vi "Image Averaging Grab (SubVI).vi"(8 "error in":errorcluster, 10 "Number of Samples":i32, 11 "Camera Session In":T1) -> (0 "error out":errorcluster, 3 "Avg Image":T2(plugin-control))   [LabVIEW 2016]
doc: "The Snap VI acquires an image and displays the image in an image control using low-level acquisition VIs. A snap is appropriate for low-speed or single-capture applications in which ease of programming is essential."
uses:
  <vilib>/userdefined/High Color/IMAQdx.ctl
  <vilib>/vision/driver/NI_Vision_Acquisition_Software.lvlib
  <resource>/objmgr/IMAQImage.rc
panel:
  in  "Standalone Mode":bool
  out "Sample #":i32
  in  "Camera Name":refnum<k21> caption="IMAQdx Session"
  out "Image":T2(plugin-control)
  # "Overview: Creates an average image from a set of collected images.\nRequirements: Vision Acquisition Software\nInstructions: \n1. Select the Camera Name.\n2. Run the VI"
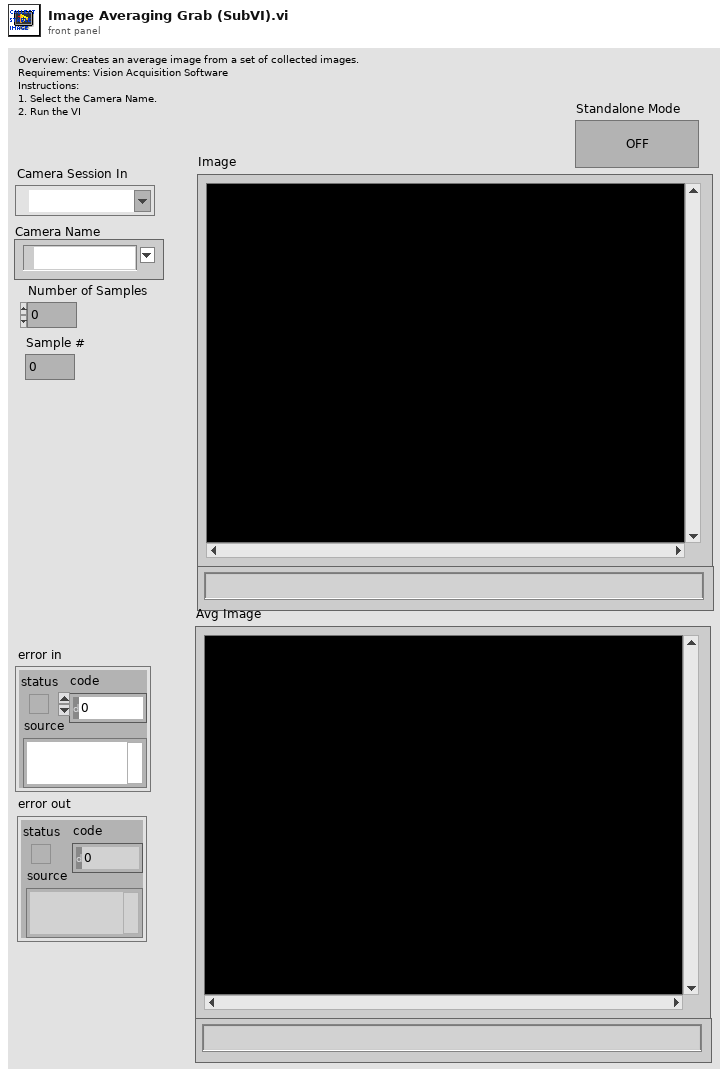
[diagram p1: front panel]
types:
  T1 = typedef "IMAQdx.ctl" = refnum<k21>
  T2 = typedef "IMAQ Image.ctl" = refnum<image>
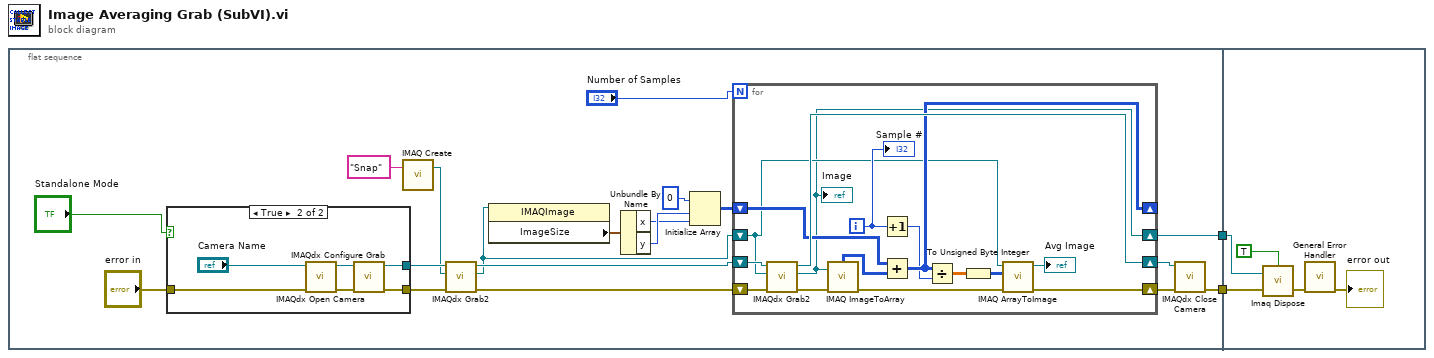
[diagram p0: block diagram]
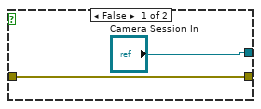
[diagram p2: hidden frame]
diagram:
  n1 = flat-sequence {
    tunnel: [w20] -> w2
    tunnel: [w9] -> w1
    tunnel: w2 -> [w50]
    tunnel: w1 -> [w48]
    frame #0 {
      n2 = case shown="True" "Standalone Mode" {
        tunnel: ["Camera Session In" w27] -> w13
        tunnel: [w22 w26] -> w11
        tunnel: "error in" -> [w22 w25]
        frame False {
        }
        frame True {
          n3 = call <vilib>:"IMAQdx Open Camera.vi"("error in"=w25, "Session In"="Camera Name") -> ("error out"=w28:errorcluster, "Session Out"=w29:T1)  [unwired: 1 in, 7 out]
          n4 = call <vilib>:"IMAQdx Configure Grab.vi"("error in"=w28, "Session In"=w29) -> ("error out"=w26:errorcluster, "Session Out"=w27:T1)  [unwired: 8 out]
        }
      }
      n5 = call "IMAQ Create"("Image Name"="Snap") -> ("New Image"=w12:T2)  [unwired: 3 in, 2 out]
      n6 = call <vilib>:"IMAQdx Grab2.vi"("error in"=w11, "Image In"=w12, "Session In"=w13) -> ("error out"=w8:errorcluster, "Image Out"=w7:T2, "Session Out"=w10:T1)  [unwired: 5 in, 1 out]
      n7 = property class="IMAQImage"(reference=w7) -> ("ImageSize"=w16:cluster{"x":i32, "y":i32})  [unwired: 1 in, 2 out]
      n8 = Unbundle By Name(w16) -> ("x"=w5:i32, "y"=w6:i32)
      n9 = Initialize Array(0 ("element"), w6, w5) -> (w15:i32[][])
      n10 = for {
        N: "Number of Samples" -> [_]
        shift-right: [w45] -> w21
        shift-left: w10 -> [w44]
        shift-right: [w33] -> w18
        shift-left: w8 -> [w43]
        shift-right: [w39] -> _
        shift-left: w15 -> [w40]
        shift-right: [w30] -> w9
        shift-left: w7 -> [w31]
        i -> [w38]
        n11 = call <vilib>:"IMAQdx Grab2.vi"("error in"=w43, "Image In"=w31, "Session In"=w44) -> ("error out"=w42:errorcluster, "Image Out"=w30:T2, "Session Out"=w45:T1)  [unwired: 5 in, 1 out]
        "Image" <- w30
        n12 = call "IMAQ ImageToArray"("error in (no error)"=w42, "Image"=w30) -> ("error out"=w34:errorcluster, "Image Pixels (U8)"=w41:u8[][])  [unwired: 2 in, 3 out]
        n13 = Increment(x=w38) -> (x+1=w37:i32)
        n14 = Add(x=w40, y=w41) -> (x+y=w39:i32[][])
        n15 = Divide(x=w39, y=w37) -> (x/y=w36:dbl[][])
        n16 = To Unsigned Byte Integer(number=w36) -> (unsigned 8bit integer=w35:u8[][])
        n17 = call "IMAQ ArrayToImage"("error in (no error)"=w34, "Image Pixels (U8)"=w35, "Image"=w31) -> ("error out"=w33:errorcluster, "Image Out"=→"Avg Image":T2)  [unwired: 7 in]
        "Sample #" <- w38
      }
      n18 = call <vilib>:"IMAQdx Close Camera.vi"("error in"=w18, "Session In"=w21) -> ("error out"=w20:errorcluster)  [unwired: 9 out]
    }
    frame #1 {
      n19 = call "Imaq Dispose"("All Images? (No)"=TRUE, "Image"=w48, "error in (no error)"=w50) -> ("error out"=w49:errorcluster)  [unwired: 3 in]
      n20 = call <vilib>:"General Error Handler.vi"("error in (no error)"=w49) -> ("error out"=→"error out":errorcluster)  [unwired: 2 in, 12 out]
    }
  }
